vi "FL fc file parser.vi"(8 "error in":errorcluster, 11 "Source File (.fc)":path) -> (0 "error out":errorcluster, 3 "fuzzy system out":T1 {"user MF interpolating polynomials"."coa_x(y) coeff" format="%.4g"; "user MF interpolating polynomials"."Area(y) coeff" format="%.4g"; "user MF interpolating polynomials"."X(y) coeff" format="%.4g"; "user MF interpolating polynomials"."Y(x) coeff" format="%.4g"; "user MF interpolating polynomials"."Y" format="%.4g"; "user MF interpolating polynomials"."X" format="%.4g"; "defuzzification method" items=["Center of Area", "Modified Center of Area", "Center of Sums", "Center of Maximum", "Mean of Maximum"]; "rules"."consequents"."Var Index" min=0; "rules"."consequents"."Cond" items=["=", "!="]; "rules"."consequents"."MF Index" min=0; "rules"."antecedents"."Var Index" min=0; "rules"."antecedents"."Cond" items=["=", "!="]; "rules"."antecedents"."MF Index" min=0; "rules"."consequent implication" items=["Minimum", "Product"]; "rules"."antecedent connective" items=["AND (Minimum)", "AND (Product)", "OR (Maximum)", "OR (Probabilistic)"]; "output variables"."MFs"."shape" items=["Triangle", "Trapezoid", "Singleton", "Sigmoid", "Gaussian", "User-Defined"]; "input variables"."MFs"."shape" items=["Triangle", "Trapezoid", "Singleton", "Sigmoid", "Gaussian", "User-Defined"]})   [LabVIEW 2013, in "NI_Fuzzy_Logic_API.lvlib"]
doc: "Open a .fc file (obsolete fuzzy logic file) and translate the information to the New Fuzzy Set datatype. This data will be used by all other Fuzzy Logic Toolkit VIs."
uses:
  <vilib>/addons/Fuzzy Logic/NI_Fuzzy_Logic_API.lvlib
  <vilib>/addons/Fuzzy Logic/TypeDefs/FL System.ctl
  <vilib>/addons/Fuzzy Logic/TypeDefs/FL Variable.ctl
  <vilib>/addons/Fuzzy Logic/TypeDefs/FL Membership Function.ctl
  <vilib>/addons/Fuzzy Logic/TypeDefs/FL Membership Function Shape.ctl
  <vilib>/addons/Fuzzy Logic/TypeDefs/FL Rule.ctl
  <vilib>/addons/Fuzzy Logic/TypeDefs/FL Antecedent.ctl
  <vilib>/addons/Fuzzy Logic/TypeDefs/FL Modifier.ctl
  <vilib>/addons/Fuzzy Logic/TypeDefs/FL Antecedent Connective.ctl
  <vilib>/addons/Fuzzy Logic/TypeDefs/FL Consequent.ctl
  <vilib>/addons/Fuzzy Logic/TypeDefs/FL Consequent Implication.ctl
  <vilib>/addons/Fuzzy Logic/TypeDefs/FL Defuzzification.ctl
  <vilib>/addons/Fuzzy Logic/TypeDefs/FL Interpolating polynomials.ctl
panel:
  out "Old Controller":T13={"Parameters"={"antecedance"=[{"ling.var."="Fuzzy-IN II", "x-min"=-10.0, "x-max"=10.0, "setarray"=[{"linguistic term"="NB", "color"=16711680, "points"=[-1.0, -1.0, -0.09999999999999998, -0.050000000000000044]}, {"linguistic term"="NS", "color"=3342438, "points"=[-0.09999999999999998, -0.050000000000000044, -0.050000000000000044, 0.0]}, {"linguistic term"="ZE", "color"=16724991, "points"=[-0.050000000000000044, 0.0, 0.0, 0.050000000000000044]}, {"linguistic term"="PS", "color"=255, "points"=[0.0, 0.050000000000000044, 0.050000000000000044, 0.10000000000000009]}, {"linguistic term"="PB", "color"=26214, "points"=[0.050000000000000044, 0.10000000000000009, 1.0, 1.0]}]}], "consequence"=[{"ling.var."="Fuzzy-OUT II", "x-min"=-10.0, "x-max"=10.0, "setarray"=[{"linguistic term"="NV", "color"=16711680, "points"=[-1.0, -1.0, -1.0, -1.0]}, {"linguistic term"="NED", "color"=3342438, "points"=[-0.5, -0.5, -0.5, -0.5]}, {"linguistic term"="NU", "color"=16724991, "points"=[0.0, 0.0, 0.0, 0.0]}, {"linguistic term"="PED", "color"=255, "points"=[0.5, 0.5, 0.5, 0.5]}, {"linguistic term"="PV", "color"=26214, "points"=[1.0, 1.0, 1.0, 1.0]}]}], "conclusions"=[0, 1, 2, 3, 4], "degree-of-support"=[1.0, 1.0, 1.0, 1.0, 1.0], "defu"=[{"inference"=0, "defumethod"=2, "modification"=TRUE, "precision"=0, "no consequence"=0, "defaultvalue"=0.0}]}, "Description"={"Info"={"Path"=path "/Mac IIsi/Work IIsi/Carsten&Stefan/Controller/Behaelter_P2.fc", "Controller Name"="Behaelter_P2.fc", "Date"="02.07.1996", "Time"="10:49 Uhr"}, "Author"="", "Description"=""}} {"Parameters"."defu"."defaultvalue" format="%.2f"; "Parameters"."degree-of-support" step=0.009999999776482582 format="%.2f"; "Parameters"."consequence"."x-min" step=0.009999999776482582 format="%.2f"; "Parameters"."consequence"."x-max" step=0.009999999776482582 format="%.2f"; "Parameters"."consequence"."setarray"."points" step=0.009999999776482582 format="%.2f"; "Parameters"."antecedance"."x-min" step=0.009999999776482582 format="%.2f"; "Parameters"."antecedance"."x-max" step=0.009999999776482582 format="%.2f"; "Parameters"."antecedance"."setarray"."points" step=0.009999999776482582 format="%.2f"}
  # "IF"
  # "THEN"
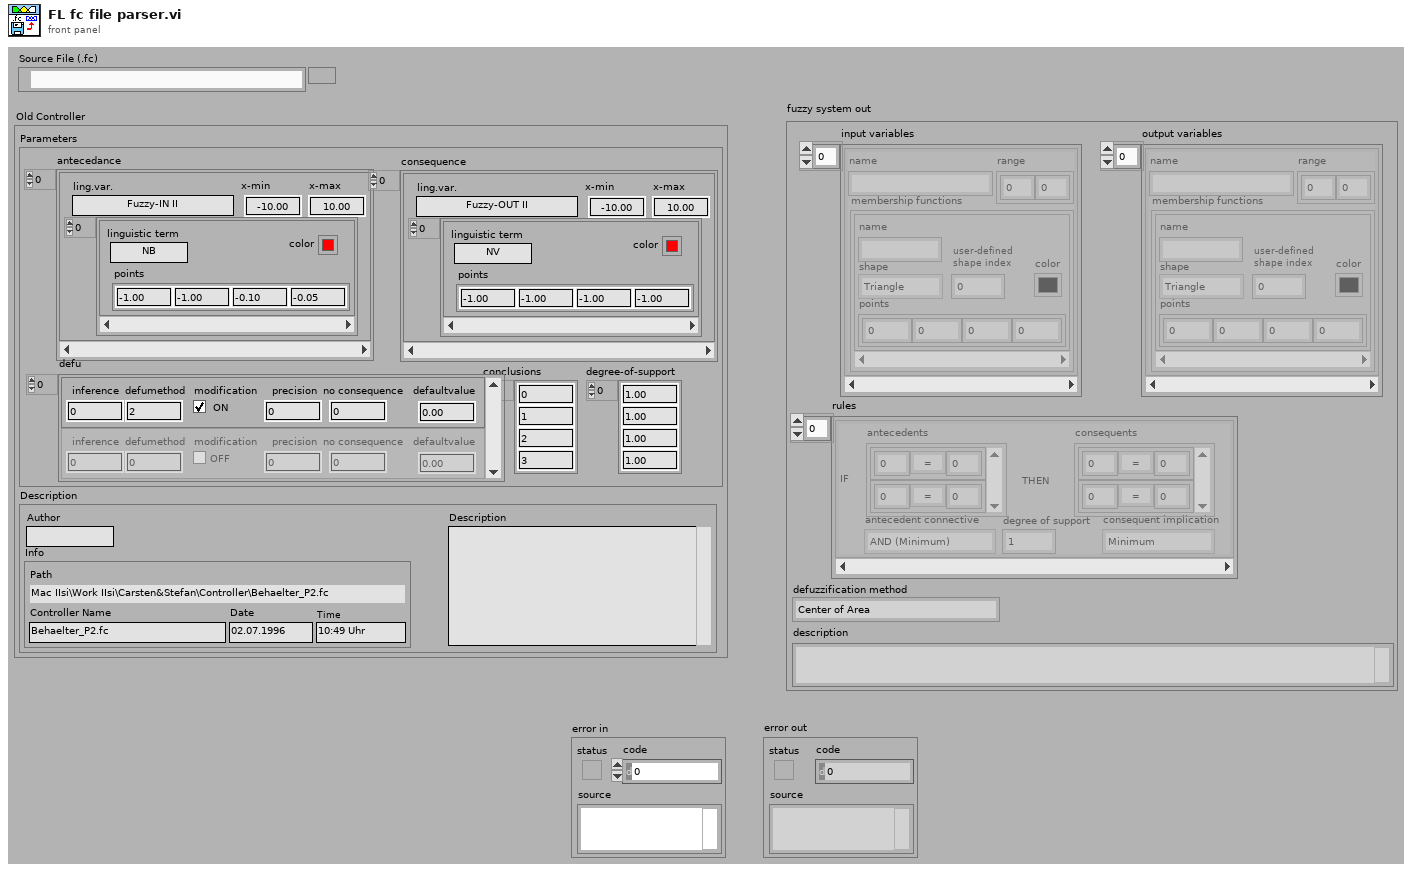
[diagram p1: front panel]
types:
  T1 = typedef "NI_Fuzzy_Logic_API.lvlib/FL System.ctl" = cluster{"input variables":T2[], "output variables":T2[], "rules":T5[], "defuzzification method":T11, "description":string, "user MF interpolating polynomials":T12[]}
  T2 = typedef "NI_Fuzzy_Logic_API.lvlib/FL Variable.ctl" = cluster{"name":string, "range":dbl[], "MFs":T3[]}
  T3 = typedef "NI_Fuzzy_Logic_API.lvlib/FL Membership Function.ctl" = cluster{"name":string, "shape":T4, "points":dbl[], "color":u32, "user-defined shape index":i32}
  T4 = typedef "NI_Fuzzy_Logic_API.lvlib/FL Membership Function Shape.ctl" = u16
  T5 = typedef "NI_Fuzzy_Logic_API.lvlib/FL Rule.ctl" = cluster{"antecedents":T6[], "antecedent connective":T8, "consequents":T9[], "consequent implication":T10, "degree of support":dbl}
  T6 = typedef "NI_Fuzzy_Logic_API.lvlib/FL Antecedent.ctl" = cluster{"Var Index":i32, "MF Index":i32, "Cond":T7}
  T7 = typedef "NI_Fuzzy_Logic_API.lvlib/FL Modifier.ctl" = u16
  T8 = typedef "NI_Fuzzy_Logic_API.lvlib/FL Antecedent Connective.ctl" = u16
  T9 = typedef "NI_Fuzzy_Logic_API.lvlib/FL Consequent.ctl" = cluster{"Var Index":i32, "MF Index":i32, "Cond":T7}
  T10 = typedef "NI_Fuzzy_Logic_API.lvlib/FL Consequent Implication.ctl" = u16
  T11 = typedef "NI_Fuzzy_Logic_API.lvlib/FL Defuzzification.ctl" = u16
  T12 = typedef "NI_Fuzzy_Logic_API.lvlib/FL Interpolating polynomials.ctl" = cluster{"X":dbl[], "Y":dbl[], "Y(x) coeff":dbl[][], "X(y) coeff":dbl[][], "Area(y) coeff":dbl[][], "coa_x(y) coeff":dbl[][]}
  T13 = cluster{"Parameters":cluster{"antecedance":cluster{"ling.var.":string, "x-min":dbl, "x-max":dbl, "setarray":cluster{"linguistic term":string, "color":u32, "points":dbl[]}[]}[], "consequence":cluster{"ling.var.":string, "x-min":dbl, "x-max":dbl, "setarray":cluster{"linguistic term":string, "color":u32, "points":dbl[]}[]}[], "conclusions":u16[], "degree-of-support":dbl[], "defu":cluster{"inference":u16, "defumethod":u16, "modification":bool, "precision":u16, "no consequence":u16, "defaultvalue":dbl}[]}, "Description":cluster{"Info":cluster{"Path":path, "Controller Name":string, "Date":string, "Time":string}, "Author":string, "Description":string}}
  T14 = enum16{"open", "replace", "create", "open or create", "replace or create", "replace or create with confirmation"}
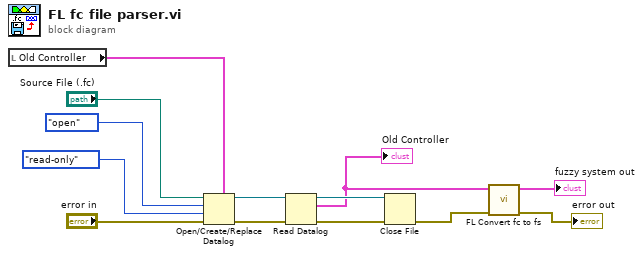
[diagram p0: block diagram]
diagram:
  n1 = local read "Old Controller"() -> (w6:T13)
  n2 = Open/Create/Replace Datalog(5:w6, 8:"error in", 9:enum16{"read/write", "read-only", "write-only"}."read-only" ("access (0:read/write)"), 10:T14."open" ("operation (0:open)"), 11:"Source File (.fc)") -> (0:w8:errorcluster, 3:w7:refnum<k1>)  [unwired: 2 out]
  n3 = Read Datalog(4:w8, 7:w7) -> (0:w9:errorcluster, 2:w1:T13, 3:w10:refnum<k1>)  [unwired: 1 out]
  "Old Controller" <- w1
  n4 = Close File(refnum=w10, error in=w9) -> (error out=w4:errorcluster)  [unwired: 1 out]
  n5 = call <vilib>:"FL Convert fc to fs.vi"("error in (no error)"=w4, "old controller in"=w1) -> ("error out"=→"error out":errorcluster, "fuzzy system out"=→"fuzzy system out":T1)  [unwired: 1 in, 7 out]
